vi "Panel.vi"(11 "DblNumericStatusEditorPanel in":refnum<class "DblNumericStatusEditorPanel.lvclass">) -> ()   [LabVIEW 2020, in "VolatusGUIControls.lvlib" / "DblNumericStatusEditorPanel.lvclass"]
uses:
  DblNumericStatusEditorPanel.lvclass
  C:/dev/lv20CE/relink/volatus-gui-controls/VolatusGUIEditorCore/ElementEditorPanel/ElementEditorPanel.lvclass
  C:/dev/lv20CE/relink/lv-oopanel/OOPanel/Panel/Panel.lvclass
  lv-oopanel/OOPanel/Panel/Basic UI State.ctl
  lv-autocomplete/AutoComplete/AutoComplete/AutoComplete.lvclass/AutoComplete.ctl
  DblNumericStatusEditorPanel.lvclass/DblNumericStatusEditorPanel.ctl
  lv-autocomplete/AutoComplete/Launch Autocomplete Handler.vi
  lv-autocomplete/AutoComplete/AutoComplete/AutoComplete.lvclass
  lv-oopanel/OOPanel/Panel/Panel.lvclass
  lv-oopanel/OOPanel/OOPanel.lvlib
  VolatusGUIEditorCore/ElementEditorPanel/ElementEditorPanel.lvclass
  VolatusGUIEditorCore/VolatusGUIEditorCore.lvlib
  C:/dev/lv20CE/relink/volatus-gui-controls/VolatusGUIControls/DblNumericStatusEditorPanel/DblNumericStatusEditorPanel.lvclass
panel:
  in  "Decimals":u8
  in  "BG Color":u32(colorbox)
  in  "Font Color":u32(colorbox)
  in  "Top":i32
  in  "Left":i32
  in  "Height":u16
  in  "Width":u16
  in  "Label Text Color":u32(colorbox) caption="Color"
  in  "Label Visible":bool caption="Visible"
  in  "Label":string
  in  "Channel":string
  # "Label"
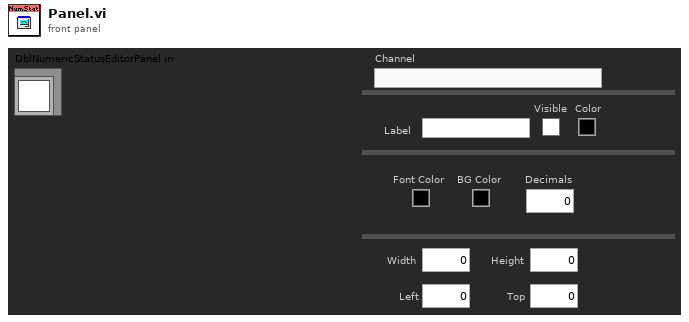
[diagram p1: front panel]
types:
  T1 = typedef "OOPanel.lvlib/Panel.lvclass/Basic UI State.ctl" = enum16{"Init", "Run", "Close"}
  T2 = typedef "VolatusGUIEditorCore.lvlib/ElementEditorPanel.lvclass/Incoming Events.ctl" = cluster{"Update Control":refnum<user-event>}
  T3 = typedef "OOPanel.lvlib/Panel.lvclass/Panel Events.ctl" = cluster{"Visbility":refnum<user-event>, "Close":refnum<user-event>}
  T4 = typedef "VolatusGUIControls.lvlib/DblNumericStatusEditorPanel.lvclass/Props.ctl" = cluster{"JSON":T5, "Label Props":T6, "Position Props":T7, "Width":u16, "Height":u16, "Numeric Text Props":T8}
  T5 = typedef "VolatusGUIControls.lvlib/DblNumericStatusEditorPanel.lvclass/JSON Props.ctl" = cluster{"Channel":string}
  T6 = typedef "VolatusGUIEditorCore.lvlib/Label Props.ctl" = cluster{"Text":string, "Text Color":u32, "Visible":bool}
  T7 = typedef "VolatusGUIEditorCore.lvlib/Position Props.ctl" = cluster{"Left":i32, "Top":i32}
  T8 = typedef "VolatusGUIEditorCore.lvlib/Numeric Text Props.ctl" = cluster{"Font Color":u32, "BG Color":u32, "Format String":string}
  T9 = typedef "OOPanel.lvlib/Visibility State.ctl" = enum16{"Idle", "Closed", "Hidden", "Visible", "Subpanel", "Hidden Subpanel"}
  T10 = cluster{"Label":string, "Label Text Color":u32, "Label Visible":bool}
  T11 = cluster{"Font Color":u32, "BG Color":u32, "Format String":string}
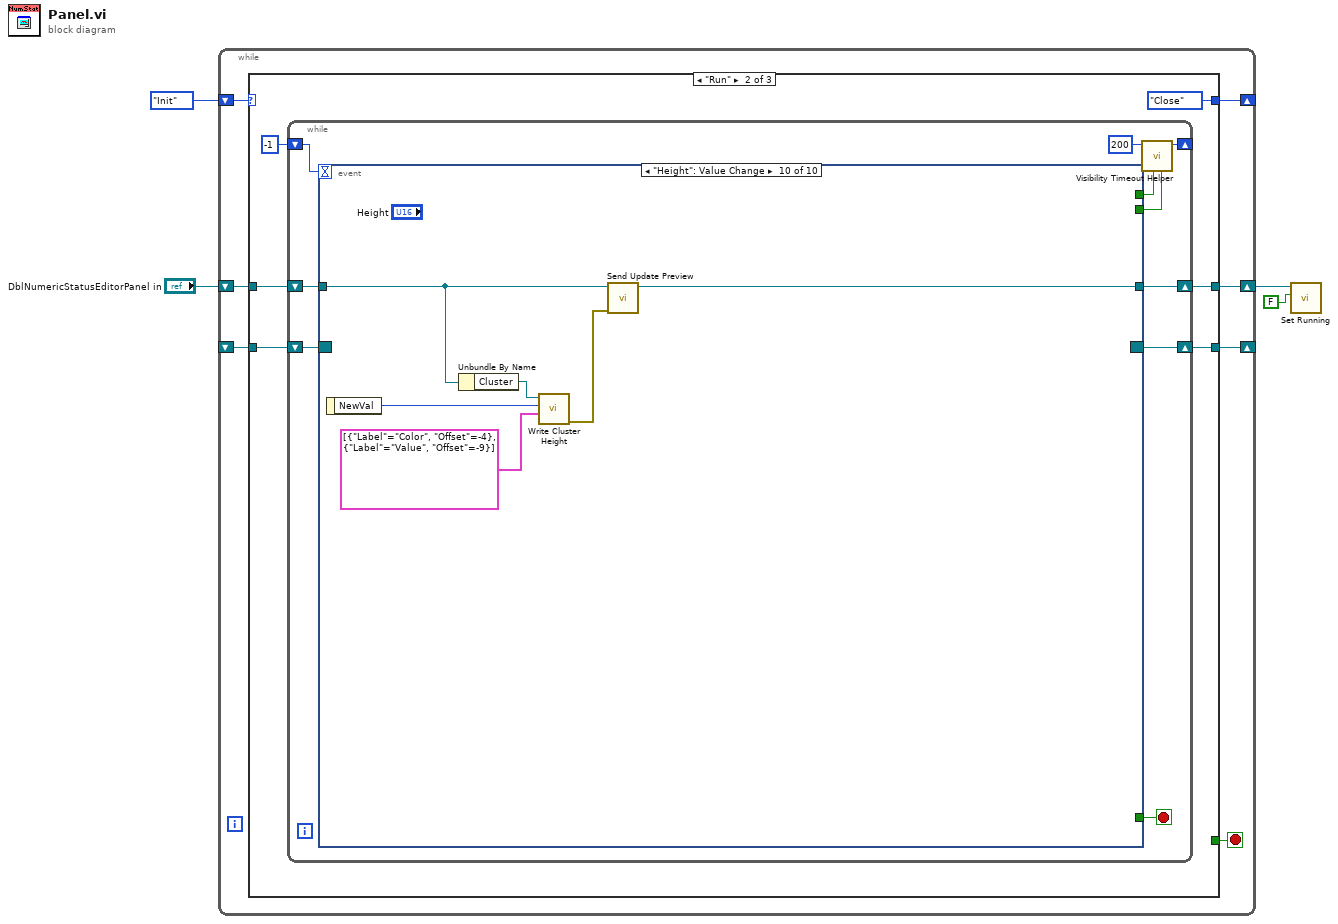
[diagram p0: block diagram]
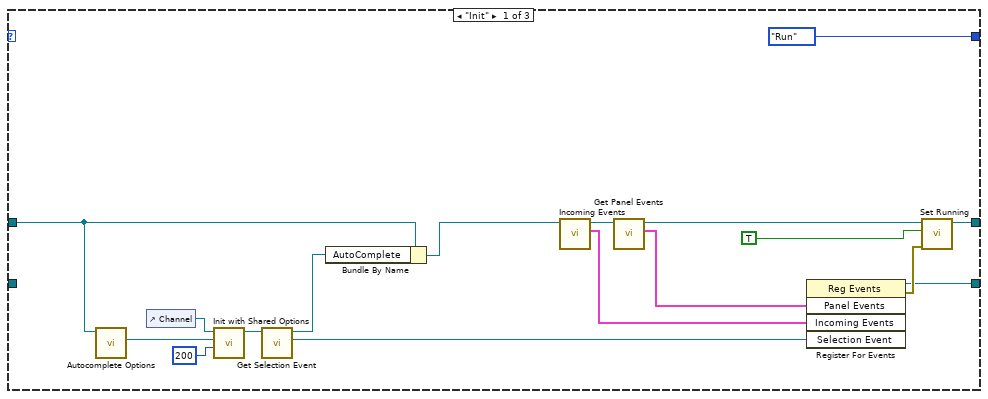
[diagram p2: hidden frame]
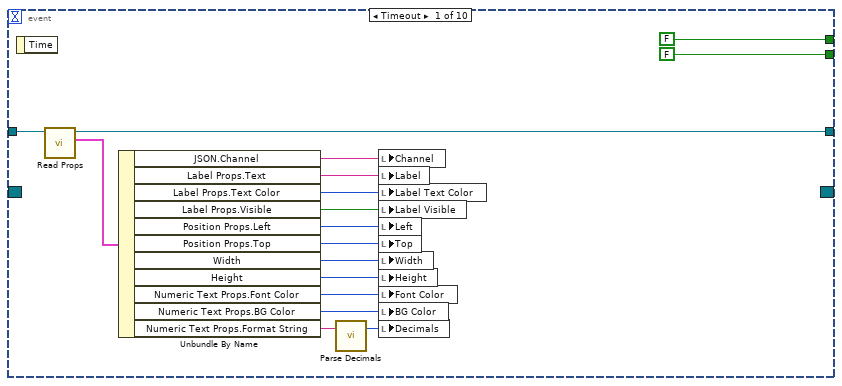
[diagram p3: hidden frame]
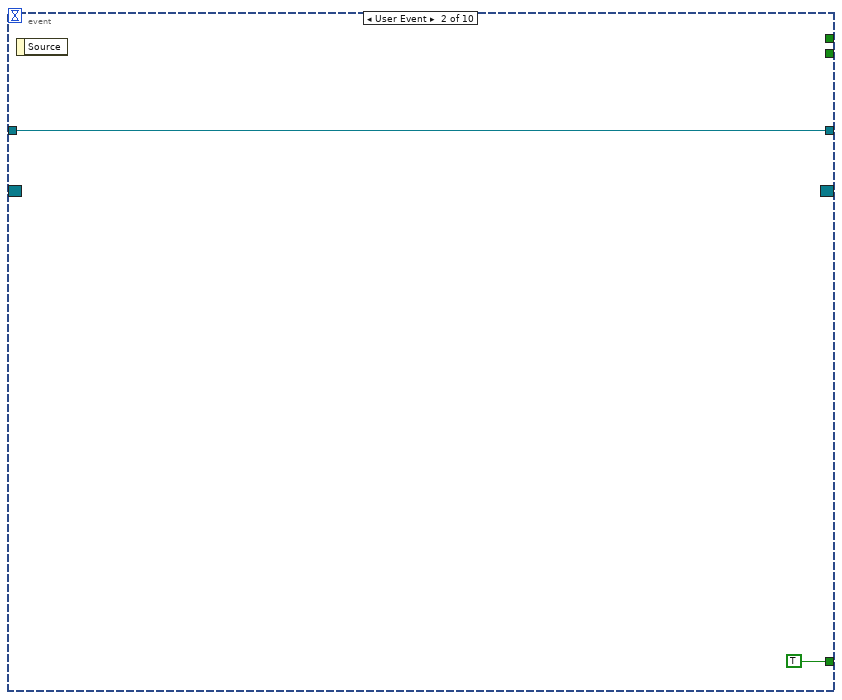
[diagram p4: hidden frame]
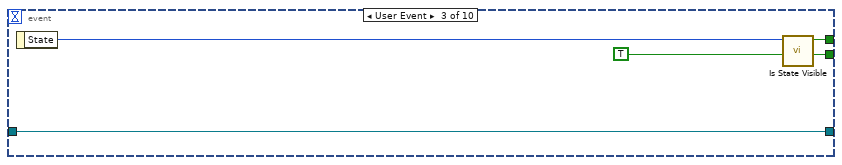
[diagram p5: hidden frame]
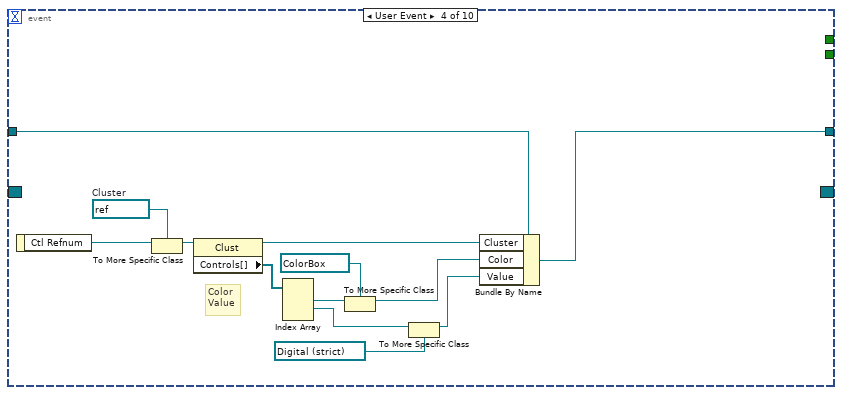
[diagram p6: hidden frame]
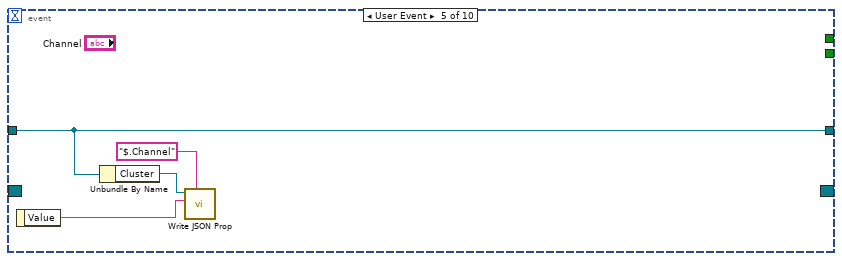
[diagram p7: hidden frame]
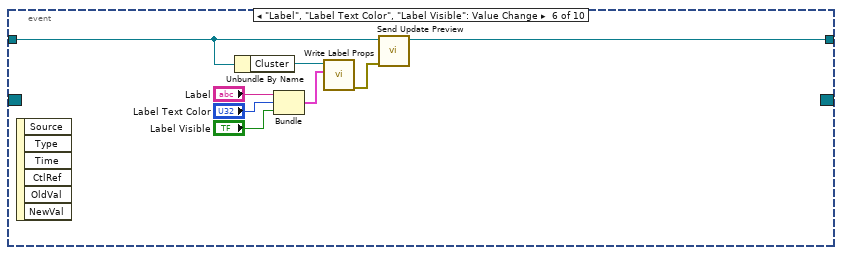
[diagram p8: hidden frame]
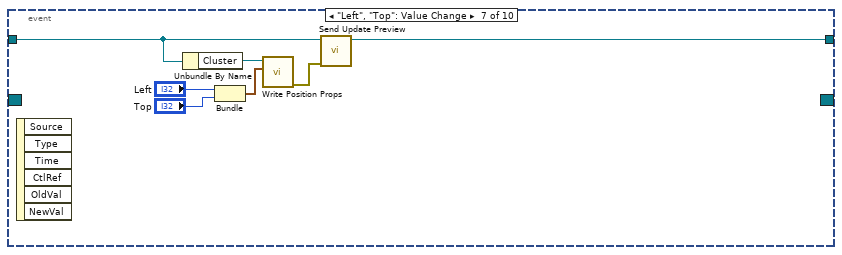
[diagram p9: hidden frame]
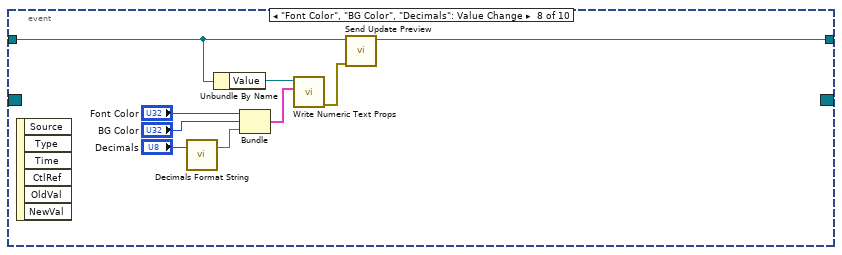
[diagram p10: hidden frame]
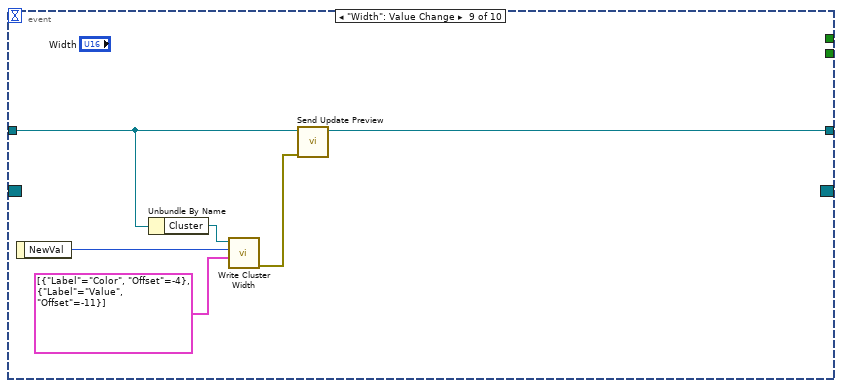
[diagram p11: hidden frame]
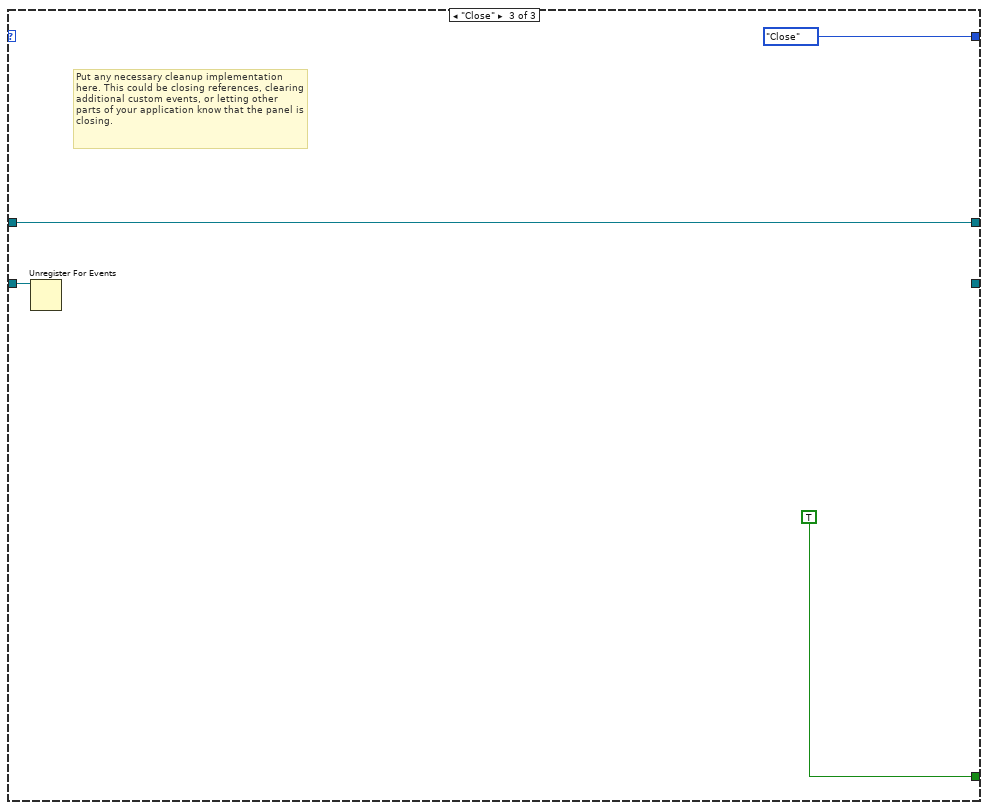
[diagram p12: hidden frame]
diagram:
  n1 = while {
    shift-right: [w10] -> _
    shift-left: _ -> [w11]
    shift-right: [w8] -> _
    shift-left: Basic_UI_State."Init" ("Basic UI State") -> [w9]
    shift-right: [w6] -> w4
    shift-left: "DblNumericStatusEditorPanel in" -> [w5]
    stop <- w7 stop-if-true
    n2 = case shown="\"Run\"" w9 {
      tunnel: w11 -> [_ w34 w122]
      tunnel: [w25 w32 _] -> w10
      tunnel: [Basic_UI_State."Run" ("Basic UI State") Basic_UI_State."Close" ("Basic UI State") Basic_UI_State."Close" ("Basic UI State")] -> w8
      tunnel: [_ _ TRUE] -> w7
      tunnel: [w24 w29 w121] -> w6
      tunnel: w5 -> [w18 w30 w121]
      frame "Init" {
        n3 = call "Autocomplete Options.vi"("ElementEditorPanel in"=w18) -> ("Autocomplete Options"=w21:refnum<class "Shared Options.lvclass">)  [unwired: 10 in]
        n4 = control-ref of="Channel"() -> (w17:refnum<vi>)
        n5 = call "Init with Shared Options.vi"("Height (200)"=i16 200, "Shared Options"=w21, "Str Refnum"=w17) -> ("AutoComplete out"=w19:refnum<class "AutoComplete.lvclass">)  [unwired: 7 in, 1 out]
        n6 = call "Get Selection Event.vi"("AutoComplete in"=w19) -> ("Selection Event"=w12:refnum<user-event>, "AutoComplete"=w13:refnum<class "AutoComplete.lvclass">)  [unwired: 9 in]
        n7 = Bundle By Name(cluster=w18, "AutoComplete"=w13) -> (w16:refnum<class "DblNumericStatusEditorPanel.lvclass">)
        n8 = call "Incoming Events.vi"("ElementEditorPanel in"=w16) -> ("Incoming Events"=w14:T2, "ElementEditorPanel out"=w15:refnum<class "DblNumericStatusEditorPanel.lvclass">)  [unwired: 9 in]
        n9 = call "Get Panel Events.vi"("Panel in"=w15) -> ("Panel Events"=w22:T3, "Panel out"=w23:refnum<class "DblNumericStatusEditorPanel.lvclass">)  [unwired: 8 in, 1 out]
        n10 = register-events(w22, w14, w12) -> (reference out=w25:refnum<event-registration>, error out=w27:errorcluster)  [unwired: 2 in]
        n11 = call "Set Running.vi"("error in (no error)"=w27, "Running"=TRUE, "Panel in"=w23) -> ("Panel out"=w24:refnum<class "DblNumericStatusEditorPanel.lvclass">)  [unwired: 7 in, 1 out]
      }
      frame "Run" {
        n12 = while {
          shift-right: [w40] -> w32
          shift-left: w34 -> [w41]
          shift-right: [w43] -> _
          shift-left: -1 ("Timeout") -> [w42]
          shift-right: [w35] -> w29
          shift-left: w30 -> [w36]
          stop <- w37 stop-if-true
          n13 = event shown="[9] \"Height\": Value Change" {
            selector: w41 -> [_ _ _ _ _ _ _ _ _ _]
            dyn-events: [_ _ _ _ _ _ _ _ _ _] -> w40
            timeout: w42 -> [_ _ _ _ _ _ _ _ _ _]
            tunnel: [FALSE _ w66 _ _ _ _ _ _ _] -> w39
            tunnel: [FALSE _ TRUE _ _ _ _ _ _ _] -> w38
            tunnel: [_ TRUE _ _ _ _ _ _ _ _] -> w37
            tunnel: w36 -> [w59 w62 w64 w69 w82 w89 w96 w103 w114 w120]
            tunnel: [w58 w62 w64 w70 w82 w86 w94 w101 w111 w117] -> w35
            event Timeout {
              n14 = event-data() -> ()  [unwired: 1 in, 1 out]
              n15 = call "Read Props.vi"("DblNumericStatusEditorPanel in"=w59) -> ("Props"=w57:T4, "DblNumericStatusEditorPanel out"=w58:refnum<class "DblNumericStatusEditorPanel.lvclass">)  [unwired: 8 in, 1 out]
              n16 = Unbundle By Name(w57) -> ("JSON.Channel"=w56:string, "Label Props.Text"=w45:string, "Label Props.Text Color"=w46:u32, "Label Props.Visible"=w47:bool, "Position Props.Left"=w48:i32, "Position Props.Top"=w49:i32, "Width"=w50:u16, "Height"=w51:u16, "Numeric Text Props.Font Color"=w52:u32, "Numeric Text Props.BG Color"=w53:u32, "Numeric Text Props.Format String"=w55:string)
              n17 = call "Parse Decimals.vi"("Format String"=w55) -> ("Decimals"=w54:u8)  [unwired: 6 in]
              n18 = local write "Channel"(w56) -> ()
              n19 = local write "Label"(w45) -> ()
              n20 = local write "Label Text Color"(w46) -> ()
              n21 = local write "Label Visible"(w47) -> ()
              n22 = local write "Left"(w48) -> ()
              n23 = local write "Top"(w49) -> ()
              n24 = local write "Width"(w50) -> ()
              n25 = local write "Height"(w51) -> ()
              n26 = local write "Font Color"(w52) -> ()
              n27 = local write "BG Color"(w53) -> ()
              n28 = local write "Decimals"(w54) -> ()
            }
            event User Event {
              n29 = event-data() -> ()  [unwired: 1 in, 1 out]
            }
            event User Event {
              n30 = event-data() -> ("State"=w67:T9)  [unwired: 1 in]
              n31 = call "Is State Visible.vi"("Visibility"=w67) -> ("Visible"=w66:bool)  [unwired: 10 in]
            }
            event User Event {
              w80 = refnum<vi> refnum  # Cluster
              # "Color\nValue"
              n32 = event-data() -> ("Ctl Refnum"=w68:refnum<vi>)  [unwired: 1 in]
              n33 = To More Specific Class(target class=w80, reference=w68) -> (specific class reference=w79:refnum<vi>)  [unwired: 1 in, 1 out]
              n34 = property class="Clust"(reference=w79) -> (reference out=w73:refnum<vi>, "Controls[]"=w78:refnum<vi>[])  [unwired: 1 in, 1 out]
              n35 = Index Array(array=w78) -> (element #1=w77:refnum<vi>, element #2=w76:refnum<vi>)  [unwired: 3 in, 1 out]
              n36 = To More Specific Class(target class=refnum<vi> refnum ("Color"), reference=w77) -> (specific class reference=w72:refnum<vi>)  [unwired: 1 in, 1 out]
              n37 = To More Specific Class(target class=refnum<vi> refnum ("Value"), reference=w76) -> (specific class reference=w71:refnum<vi>)  [unwired: 1 in, 1 out]
              n38 = Bundle By Name(cluster=w69, "Cluster"=w73, "Color"=w72, "Value"=w71) -> (w70:refnum<class "DblNumericStatusEditorPanel.lvclass">)
            }
            event User Event {
              n39 = event-data() -> ("Value"=w81:string)  [unwired: 1 in]
              n40 = Unbundle By Name(w82) -> ("Cluster"=w84:refnum<vi>)
              n41 = call "Write JSON Prop.vi"("JSON Path"="$.Channel" ("$Path or Item Name"), "Value"=w81, "Ctl Refnum in"=w84) -> ()  [unwired: 7 in, 2 out]
            }
            event "Label", "Label Text Color", "Label Visible": Value Change {
              n42 = event-data() -> ()  [unwired: 1 in, 6 out]
              n43 = Unbundle By Name(w89) -> ("Cluster"=w88:refnum<vi>)
              n44 = Bundle("Label"="Label", "Label Text Color"="Label Text Color", "Label Visible"="Label Visible") -> (w87:T10)  [unwired: 1 in]
              n45 = call "Write Label Props.vi"("Label Props"=w87, "Ctl Refnum in"=w88) -> ("error out"=w85:errorcluster)  [unwired: 8 in, 1 out]
              n46 = call "Send Update Preview.vi"("error in (no error)"=w85, "ElementEditorPanel in"=w89) -> ("ElementEditorPanel out"=w86:refnum<class "DblNumericStatusEditorPanel.lvclass">)  [unwired: 8 in, 1 out]
            }
            event "Left", "Top": Value Change {
              n47 = event-data() -> ()  [unwired: 1 in, 6 out]
              n48 = Unbundle By Name(w96) -> ("Cluster"=w95:refnum<vi>)
              n49 = Bundle("Left"="Left", "Top"="Top") -> (w97:cluster{"Left":i32, "Top":i32})  [unwired: 1 in]
              n50 = call "Write Position Props.vi"("Position Props"=w97, "Ctl Refnum in"=w95) -> ("error out"=w93:errorcluster)  [unwired: 8 in, 1 out]
              n51 = call "Send Update Preview.vi"("error in (no error)"=w93, "ElementEditorPanel in"=w96) -> ("ElementEditorPanel out"=w94:refnum<class "DblNumericStatusEditorPanel.lvclass">)  [unwired: 8 in, 1 out]
            }
            event "Font Color", "BG Color", "Decimals": Value Change {
              n52 = event-data() -> ()  [unwired: 1 in, 6 out]
              n53 = call "Decimals Format String.vi"("Decimals"="Decimals") -> ("Format String"=w105:string)  [unwired: 6 in]
              n54 = Unbundle By Name(w103) -> ("Value"=w102:refnum<vi>)
              n55 = Bundle("Font Color"="Font Color", "BG Color"="BG Color", "Format String"=w105) -> (w104:T11)  [unwired: 1 in]
              n56 = call "Write Numeric Text Props.vi"("Numeric Text Props"=w104, "Control in"=w102) -> ("error out"=w100:errorcluster)  [unwired: 8 in, 1 out]
              n57 = call "Send Update Preview.vi"("error in (no error)"=w100, "ElementEditorPanel in"=w103) -> ("ElementEditorPanel out"=w101:refnum<class "DblNumericStatusEditorPanel.lvclass">)  [unwired: 8 in, 1 out]
            }
            event "Width": Value Change {
              n58 = event-data() -> ("NewVal"=w112:u16)  [unwired: 1 in]
              n59 = Unbundle By Name(w114) -> ("Cluster"=w113:refnum<vi>)
              n60 = call "Write Cluster Width.vi"("Nested Offsets (None)"=cluster{"Label":string, "Offset":i32}[] [{"Label"="Color", "Offset"=-4}, {"Label"="Value", "Offset"=-11}], "Width"=w112, "Cluster in"=w113) -> ("error out"=w110:errorcluster)  [unwired: 7 in, 1 out]
              n61 = call "Send Update Preview.vi"("error in (no error)"=w110, "ElementEditorPanel in"=w114) -> ("ElementEditorPanel out"=w111:refnum<class "DblNumericStatusEditorPanel.lvclass">)  [unwired: 8 in, 1 out]
            }
            event "Height": Value Change {
              n62 = event-data() -> ("NewVal"=w118:u16)  [unwired: 1 in]
              n63 = Unbundle By Name(w120) -> ("Cluster"=w119:refnum<vi>)
              n64 = call "Write Cluster Height.vi"("Nested Offsets (None)"=cluster{"Label":string, "Offset":i32}[] [{"Label"="Color", "Offset"=-4}, {"Label"="Value", "Offset"=-9}], "Height"=w118, "Cluster in"=w119) -> ("error out"=w116:errorcluster)  [unwired: 7 in, 1 out]
              n65 = call "Send Update Preview.vi"("error in (no error)"=w116, "ElementEditorPanel in"=w120) -> ("ElementEditorPanel out"=w117:refnum<class "DblNumericStatusEditorPanel.lvclass">)  [unwired: 8 in, 1 out]
            }
          }
          n66 = call "Visibility Timeout Helper.vi"("Update?"=w38, "Use Timeout?"=w39, "Visible Timeout mS"=200) -> ("Timeout"=w43:i32)  [unwired: 8 in]
        }
      }
      frame "Close" {
        # "Put any necessary cleanup implementation here. This could be closing references, clearing additional custom events, or letting other parts of your application know that the panel is closing."
        n67 = Unregister For Events(event registration refnum=w122) -> ()  [unwired: 1 in, 1 out]
      }
    }
  }
  n68 = call "Set Running.vi"("Running"=FALSE, "Panel in"=w4) -> ()  [unwired: 8 in, 2 out]
